vi "Reset Feature Extraction.vi"(8 "error in (no error)":errorcluster) -> (0 "error out":errorcluster)   [LabVIEW 2013]
panel:
  in  "Non-tip Data File":path=path "C:/Users/Andrew/Documents/Apatite to Zircon Code/Track Finding/Non-tip Data.csv"
  in  "Tip Data File":path=path "C:/Users/Andrew/Documents/Apatite to Zircon Code/Track Finding/Tip Data.csv"
  in  "Non-tips Root":path=path "C:/Users/Andrew/Documents/Apatite to Zircon Code/Track Finding/Tip Images/Non-Tips"
  in  "Tips Root":path=path "C:/Users/Andrew/Documents/Apatite to Zircon Code/Track Finding/Tip Images/Tips"
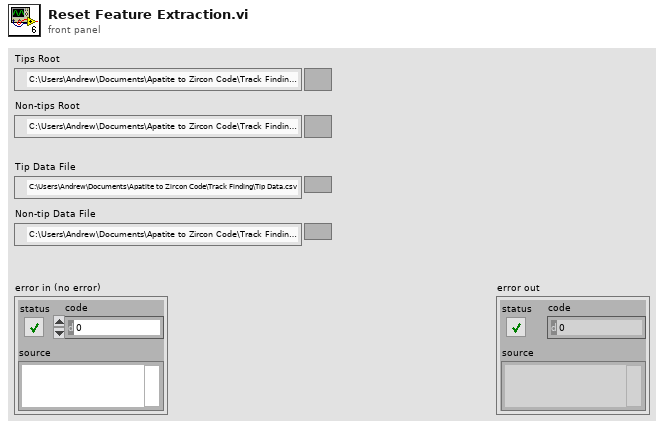
[diagram p1: front panel]
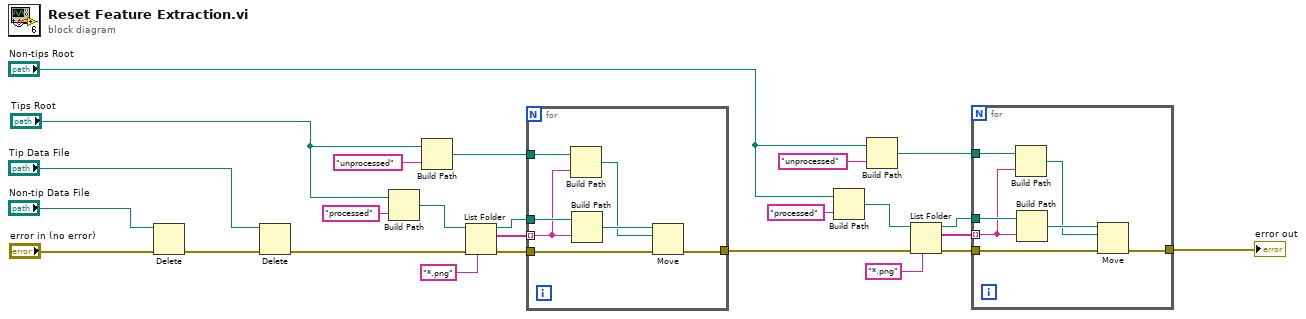
[diagram p0: block diagram]
diagram:
  n1 = Delete(path (use dialog)="Non-tip Data File", error in="error in (no error)") -> (error out=w24:errorcluster)  [unwired: 3 in, 2 out]
  n2 = Delete(path (use dialog)="Tip Data File", error in=w24) -> (error out=w15:errorcluster)  [unwired: 3 in, 2 out]
  n3 = Build Path(base path="Tips Root", name or relative path="processed") -> (appended path=w19:path)
  n4 = Build Path(base path="Tips Root", name or relative path="unprocessed") -> (appended path=w16:path)
  n5 = List Folder(path=w19, pattern="*.png", error in=w15) -> (path out=w17:path, filenames=w18:string[], error out=w20:errorcluster)  [unwired: 1 in, 1 out]
  n6 = for {
    tunnel: w20 -> [w26]
    tunnel: w18 -> [w29] mode=indexing
    tunnel: w17 -> [w32]
    tunnel: w16 -> [w30]
    tunnel: [w27] -> w3
    n7 = Build Path(base path=w30, name or relative path=w29) -> (appended path=w28:path)
    n8 = Build Path(base path=w32, name or relative path=w29) -> (appended path=w31:path)
    n9 = Move(source path=w31, error in=w26, 10:w28) -> (error out=w27:errorcluster)  [unwired: 2 in, 2 out]
  }
  n10 = Build Path(base path="Non-tips Root", name or relative path="processed") -> (appended path=w9:path)
  n11 = Build Path(base path="Non-tips Root", name or relative path="unprocessed") -> (appended path=w6:path)
  n12 = List Folder(path=w9, pattern="*.png", error in=w3) -> (path out=w7:path, filenames=w8:string[], error out=w10:errorcluster)  [unwired: 1 in, 1 out]
  n13 = for {
    tunnel: w10 -> [w33]
    tunnel: w8 -> [w36] mode=indexing
    tunnel: w7 -> [w39]
    tunnel: w6 -> [w37]
    tunnel: [w34] -> w1
    n14 = Build Path(base path=w37, name or relative path=w36) -> (appended path=w35:path)
    n15 = Build Path(base path=w39, name or relative path=w36) -> (appended path=w38:path)
    n16 = Move(source path=w38, error in=w33, 10:w35) -> (error out=w34:errorcluster)  [unwired: 2 in, 2 out]
  }
  "error out" <- w1
